vi "0~1随机数发生器1D（dbl)(白噪声）.vi"(8 "Error In":errorcluster caption="错误输入", 10 "samples":i32=128 caption="Length") -> (0 "Error Out":errorcluster caption="错误输出", 3 "Rand(0-1)":dbl[](array[numeric]))   [LabVIEW 2013]
uses:
  <vilib>/Analysis/NI_AALBase.lvlib
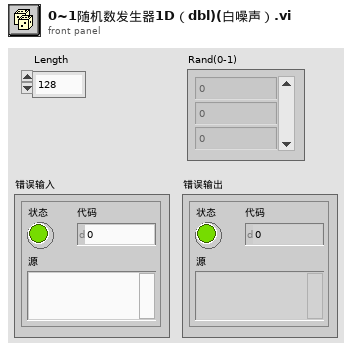
[diagram p1: front panel]
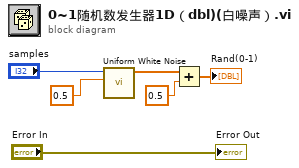
[diagram p0: block diagram]
diagram:
  n1 = call <vilib>:"Uniform White Noise.vi"("amplitude"=0.5, "samples"="samples") -> ("uniform white noise"=w4:dbl[])  [unwired: 8 in, 1 out]
  n2 = Add(x=w4, y=0.5 ("amplitude")) -> (x+y=→"Rand(0-1)":dbl[])
  "Error Out" <- "Error In"
